vi "Create PPL Build Spec.vi"(8 "error in (no error)":errorcluster, 10 "measurement plug-in name":string, 11 "project refnum":refnum<vi>) -> (0 "error out":errorcluster, 2 "measurement UI built path":path)   [LabVIEW 2020, in "MeasurementService Editor.lvlib"]
uses:
  MeasurementService Editor.lvlib
  <vilib>/AppBuilder/AB_API/PPL/NI_AB_API_PPL.lvclass
  <vilib>/Utility/LVLibp/NI_PackedLibraryUtility.lvlib
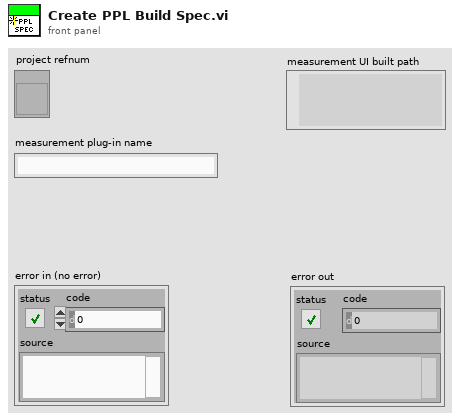
[diagram p1: front panel]
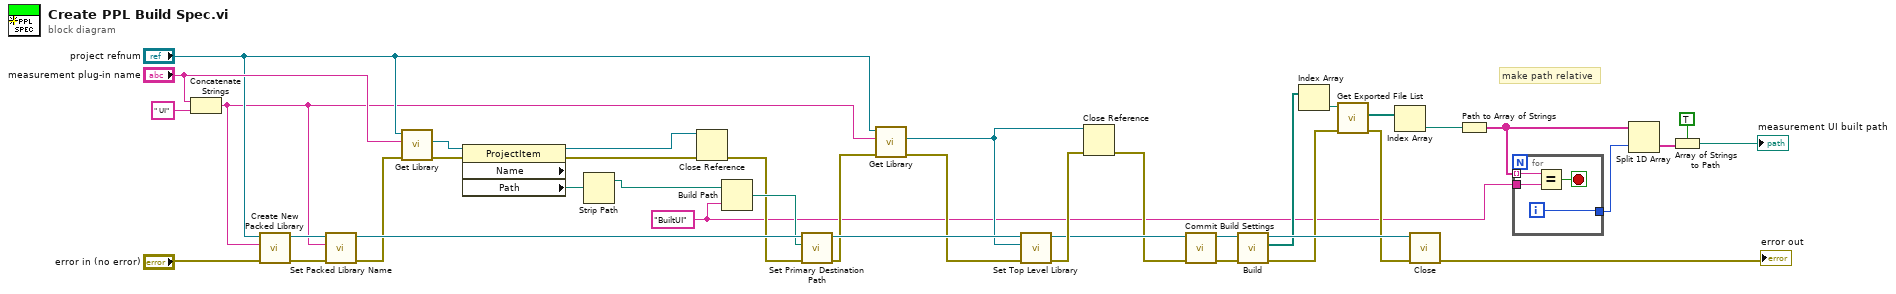
[diagram p0: block diagram]
diagram:
  w1 = "BuiltUI" ("y")
  # "make path relative"
  n1 = Concatenate Strings("measurement plug-in name", " UI" ("string")) -> (w23:string)
  n2 = call <vilib>:"Create New Packed Library.vi"("error in (no error)"="error in (no error)", "Build specification name"=w23, "Project Refnum"="project refnum") -> ("error out"=w39:errorcluster, "PPL out"=w38:refnum<class "NI_AB_API_PPL.lvclass">)  [unwired: 7 in]
  n3 = call-dynamic "Set Packed Library Name.vi"("error in (no error)"=w39, "Packed library name"=w23, "PPL in"=w38) -> ("error out"=w32:errorcluster, "PPL out"=w34:refnum<class "NI_AB_API_PPL.lvclass">)  [unwired: 7 in]
  n4 = call "Get Library.vi"("error in (no error)"=w32, "library name"="measurement plug-in name", "project in"="project refnum") -> ("error out"=w30:errorcluster, "library item"=w31:refnum<vi>)  [unwired: 6 in, 1 out]
  n5 = property class="ProjectItem" props=["Name", "Path"](reference=w31, error in=w30) -> (reference out=w27:refnum<vi>, error out=w28:errorcluster, "Path"=w17:path)  [unwired: 1 out]
  n6 = Strip Path(path=w17) -> (stripped path=w16:path)  [unwired: 1 out]
  n7 = Close Reference(reference=w27, error in (no error)=w28) -> (error out=w26:errorcluster)
  n8 = Build Path(base path=w16, name or relative path=w1) -> (appended path=w29:path)
  n9 = call-dynamic "Set Primary Destination Path.vi"("error in (no error)"=w26, "Destination path"=w29, "Build in"=w34) -> ("error out"=w25:errorcluster, "Build out"=w35:refnum<class "NI_AB_API_PPL.lvclass">)  [unwired: 7 in]
  n10 = call "Get Library.vi"("error in (no error)"=w25, "library name"=w23, "project in"="project refnum") -> ("error out"=w22:errorcluster, "library item"=w20:refnum<vi>)  [unwired: 6 in, 1 out]
  n11 = call-dynamic "Set Top Level Library.vi"("error in (no error)"=w22, "ProjectItem Refnum"=w20, "PPL in"=w35) -> ("error out"=w21:errorcluster, "PPL out"=w19:refnum<class "NI_AB_API_PPL.lvclass">)  [unwired: 7 in]
  n12 = Close Reference(reference=w20, error in (no error)=w21) -> (error out=w18:errorcluster)
  n13 = call-dynamic "Commit Build Settings.vi"("error in (no error)"=w18, "PPL in"=w19) -> ("error out"=w15:errorcluster, "PPL out"=w13:refnum<class "NI_AB_API_PPL.lvclass">)  [unwired: 8 in]
  n14 = call-dynamic "Build.vi"("error in (no error)"=w15, "PPL in"=w13) -> ("error out"=w12:errorcluster, "GeneratedFiles"=w11:path[], "PPL out"=w14:refnum<class "NI_AB_API_PPL.lvclass">)  [unwired: 6 in, 1 out]
  n15 = Index Array(array=w11) -> (element=w10:path)  [unwired: 1 in]
  n16 = call <vilib>:"Get Exported File List.vi"("error in (no error)"=w12, "packed library path"=w10) -> ("error out"=w8:errorcluster, "paths"=w9:path[])  [unwired: 7 in, 1 out]
  n17 = Index Array(array=w9) -> (element=w3:path)  [unwired: 1 in]
  n18 = call-dynamic "Close.vi"("error in (no error)"=w8, "DLL in"=w14) -> ("error out"=→"error out":errorcluster)  [unwired: 9 in]
  n19 = Path to Array of Strings(0:w3) -> (2:w7:string[])  [unwired: 1 out]
  n20 = for {
    tunnel: w7 -> [w44] mode=indexing
    tunnel: w1 -> [w43]
    tunnel: [w41] -> w6
    i -> [w41]
    stop <- w42 stop-if-true
    n21 = Equal?(x=w44, y=w43) -> (x = y?=w42:bool)
  }
  n22 = Split 1D Array(array=w7, index=w6) -> (second subarray=w5:string[])  [unwired: 1 out]
  n23 = Array of Strings to Path(0:w5, 1:TRUE ("relative")) -> (2:→"measurement UI built path":path)
